vi "Drive Path Logging Data.vi"() -> ()   [LabVIEW 2016]
panel:
  out "In Command Drive Path":bool
  in  "Drive Path Play State":string
  out "Right Sensor Velocity":dbl
  out "Right Sensor Position":dbl
  out "Right Mot Prof Active Position":dbl
  out "Right Mot Prof Active Velocity":dbl
  out "Left Sensor Velocity":dbl
  out "Left Sensor Position":dbl
  out "Left Mot Prof Active Position":dbl
  out "Left Mot Prof Active Velocity":dbl
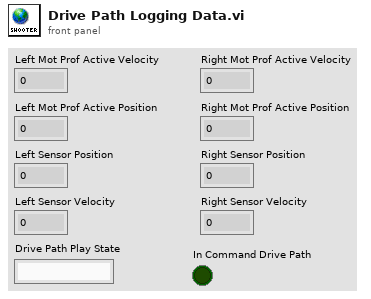
[diagram p1: front panel]
diagram:
